vi "Data Write.vi"(7 "Retry Attempts (0)":i32 min=0, 8 "error in (no error)":errorcluster, 10 "Command":string, 11 "VISA Refnum in":refnum<visa-resource-name>) -> (0 "error out":errorcluster, 3 "VISA Refnum out":refnum<visa-resource-name>)   [LabVIEW 2020, in "ChromTech Series III Pump.lvlib"]
doc: "Performs a VISA Write to the given VISA port with the given command. The write action will be retried upon failure up to N times, where N is the Retry Attempts given, where N >= 0. Values less than zero will be treated as zero. The first wait time is 1 second, which doubles in subsequent retry wait times, similar to TCP communications prior to any segments being received.\n\nFor example, attempt 1 (0 retries) = 1 second wait; attempt 2 (1 retry) = 2 second wait; attempt 3 (2 retries) = 4 second wait. The number of seconds waited on a given retry attempt can be represented with the formula 2^n, where n is the number of retries attempted."
uses:
  <instrlib>/RxnRover/ChromtechSeriesIIIDriver/ChromTech Series III Pump.lvlib
  <vilib>/Utility/sysdir.llb/System Directory Type.ctl
panel:
  out "Retries":i32
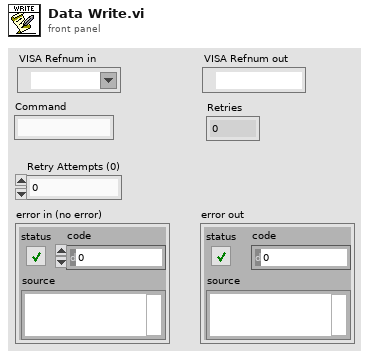
[diagram p1: front panel]
types:
  T1 = typedef "System Directory Type.ctl" = i32
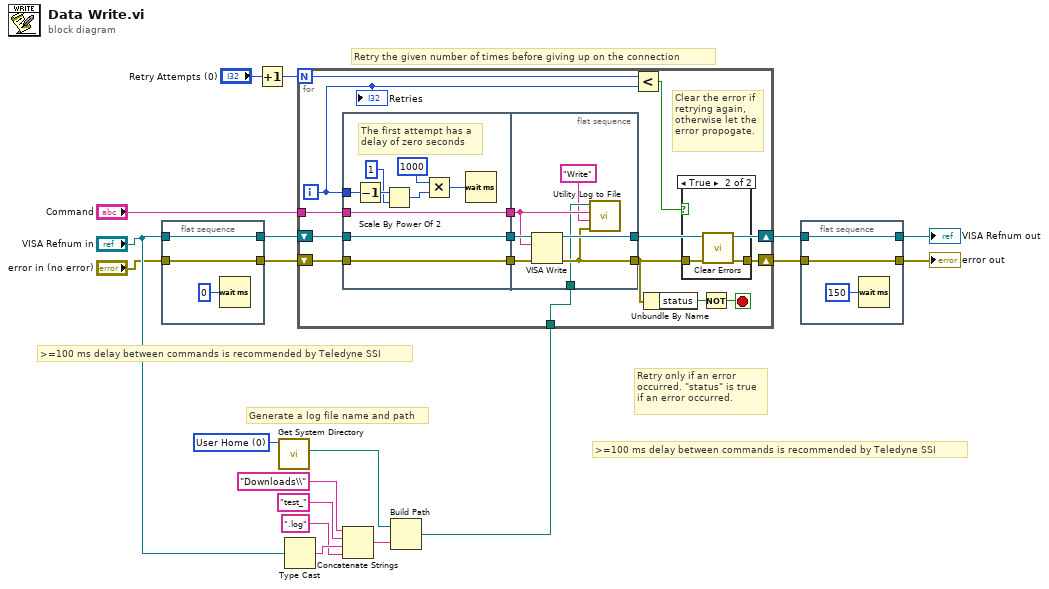
[diagram p0: block diagram]
diagram:
  w16 = T1 0 items=["User Home"=0, "User Desktop"=1, "User Documents"=2, "User Application Data"=3, "User Preferences"=4, "User Temporary"=5, "Public Documents"=6, "Public Application Data"=7, "Public Preferences"=8, "Public Cache"=13, "System Core Libraries"=9, "System Installed Libraries"=10, "Application Files"=11, "Boot Volume Root"=12] ("system directory type")
  # ">=100 ms delay between commands is recommended by Teledyne SSI"
  # ">=100 ms delay between commands is recommended by Teledyne SSI"
  # "Retry only if an error\noccurred. \"status\" is true\nif an error occurred."
  # "Retry the given number of times before giving up on the connection"
  # "Generate a log file name and path"
  n1 = flat-sequence {
    tunnel: "error in (no error)" -> [w22]
    tunnel: "VISA Refnum in" -> [w21]
    tunnel: [w21] -> w8
    tunnel: [w22] -> w5
    frame #0 {
      n2 = Wait (ms)(milliseconds to wait=u32 0) -> ()  [unwired: 1 out]
    }
  }
  n3 = Increment(x="Retry Attempts (0)") -> (x+1=w9:i32)
  n4 = call <vilib>:"Get System Directory.vi"("system directory type"=w16) -> ("system directory"=w12:path)  [unwired: 10 in]
  n5 = Type Cast(x="VISA Refnum in") -> (*(type *) &x=w18:string)  [unwired: 1 in]
  n6 = Concatenate Strings("Downloads\\", "test_", w18, ".log") -> (w13:string)
  n7 = Build Path(base path=w12, name or relative path=w13) -> (appended path=w11:path)
  n8 = for {
    N: w9 -> [w24]
    tunnel: "Command" -> [w34]
    tunnel: w11 -> [w30]
    shift-right: [w37] -> w4
    shift-left: w8 -> [w36]
    shift-right: [w26] -> w3
    shift-left: w5 -> [w35]
    i -> [w23]
    stop <- w27 stop-if-true
    # "Clear the error if\nretrying again,\notherwise let the\nerror propogate."
    n9 = flat-sequence {
      tunnel: w34 -> [w47]
      tunnel: w35 -> [w48]
      tunnel: w36 -> [w49]
      tunnel: [w49] -> w33
      tunnel: [w48] -> w32
      tunnel: [w47] -> w31
      tunnel: w23 -> [w46]
      tunnel: [w56] -> w37
      tunnel: [w53] -> w29
      tunnel: w30 -> [w51]
      tunnel: w33 -> [w55]
      tunnel: w32 -> [w54]
      tunnel: w31 -> [w52]
      frame #0 {
        # "The first attempt has a \ndelay of zero seconds"
        n10 = Decrement(x=w46) -> (x-1=w42:i32)
        n11 = Scale By Power Of 2(n=w42, x=1) -> (x*2^n=w45:i32)
        n12 = Multiply(x=1000, y=w45) -> (x*y=w43:i32)
        n13 = Wait (ms)(milliseconds to wait=w43) -> ()  [unwired: 1 out]
      }
      frame #1 {
        n14 = VISA Write(VISA resource name=w55, write buffer=w52, error in (no error)=w54) -> (VISA resource name out=w56:refnum<visa-resource-name>, error out=w53:errorcluster)  [unwired: 1 out]
        n15 = call <instrlib>:"Utility Log to File.vi"("error in (no error)"=w53, "Additional Notes"="Write", "Command"=w52, "Log File Path"=w51) -> ()  [unwired: 7 in, 1 out]
      }
    }
    n16 = Less?(x=w24, y=w23) -> (x < y?=w25:bool)
    n17 = Unbundle By Name(w29) -> ("status"=w28:bool)
    n18 = case shown="True" w25 {
      tunnel: w29 -> [w38 w40]
      tunnel: [w38 w39] -> w26
      frame False {
      }
      frame True {
        n19 = call <vilib>:"Clear Errors.vi"("error in (no error)"=w40) -> ("error out"=w39:errorcluster)  [unwired: 5 in, 1 out]
      }
    }
    n20 = Not(x=w28) -> (.not. x?=w27:bool)
    "Retries" <- w23
  }
  n21 = flat-sequence {
    tunnel: w3 -> [w59]
    tunnel: w4 -> [w58]
    tunnel: [w58] -> w1
    tunnel: [w59] -> w2
    frame #0 {
      n22 = Wait (ms)(milliseconds to wait=u32 150) -> ()  [unwired: 1 out]
    }
  }
  "VISA Refnum out" <- w1
  "error out" <- w2
